vi "Arms Command.vi"(11 "Numeric":dbl) -> (1 "RightArmMotorCmd":dbl(graph), 2 "Right Arm Min Limit":bool, 3 "Right Arm Max Limit":bool, 4 "LeftArmMotorCmd":dbl(graph), 5 "Left Arm Max Limit":bool, 6 "Left Arm Min Limit":bool)   [LabVIEW 2017]
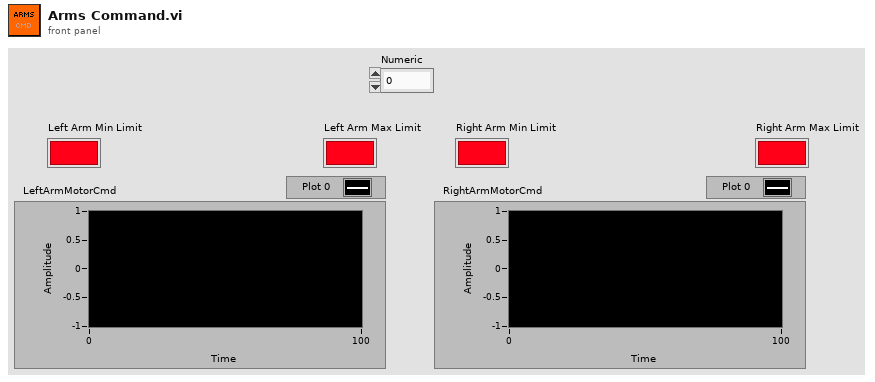
[diagram p1: front panel]
types:
  T1 = enum16{"initialize", "read", "write", "write all"}
  T2 = typedef "DioDisplayALB.ctl" = cluster{"DIO 0-LiftMinLimitSwitch":bool, "DIO 1-LiftMaxLimitSwitch":bool, "DIO 2-LiftArmMinLimitSwitch":bool, "DIO 3-LiftArmMaxLimitSwitch":bool, "DIO 4-RightArmMaxLimitSwitch":bool, "DIO 5-RightArmMinLimitSwitch":bool, "DIO 6-LeftArmMaxLimitSwitch":bool, "DIO 7-LeftArmMinLimitSwitch":bool, "DIO 8":bool, "DIO 9":bool}
  T3 = typedef "WPI_MotorControlDeviceRef.ctl" = cluster{"DeviceStatus":errorcluster, "Type":T4, "PWM":cluster{"PWM Channel":T5, "DeadBand":T6}, "CAN":cluster{"Device Number":u8, "SetOutput VI Ref":variant, "GetOutput VI Ref":variant, "Enable VI Ref":variant, "Disable VI Ref":variant, "Data":variant}, "Invert":bool, "DIO PWM":cluster{"PWM \"Enable\" Channel":T5, "DIOChannel":T7, "PWM Rate":dbl}}
  T4 = typedef "WPI_MotorControlType.ctl" = enum16{"PWM", "CAN", "DIO PWM"}
  T5 = typedef "FPGA_DIOPWMChannel.ctl" = enum8{"PWM 0", "PWM 1", "PWM 2", "PWM 3", "PWM 4", "PWM 5", "PWM 6", "PWM 7", "PWM 8", "PWM 9", "PWM MXP 0", "PWM MXP 1", "PWM MXP 2", "PWM MXP 3", "PWM MXP 4", "PWM MXP 5", "PWM MXP 6", "PWM MXP 7", "PWM MXP 8", "PWM MXP 9", "Invalid"}
  T6 = typedef "WPI_PWMDeadband.ctl" = cluster{"Name":string, "maxPositivePwm":i32, "minPositivePwm":i32, "centerPwm":i32, "maxNegativePwm":i32, "minNegativePwm":i32, "angularRange":u16}
  T7 = typedef "FPGA_DIOChannel.ctl" = enum8{"DIO 0", "DIO 1", "DIO 2", "DIO 3", "DIO 4", "DIO 5", "DIO 6", "DIO 7", "DIO 8", "DIO 9", "DIO MXP 0", "DIO MXP 1", "DIO MXP 2", "DIO MXP 3", "DIO MXP 4", "DIO MXP 5", "DIO MXP 6", "DIO MXP 7", "DIO MXP 8", "DIO MXP 9", "DIO MXP 10", "DIO MXP 11", "DIO MXP 12", "DIO MXP 13", "DIO MXP 14", "DIO MXP 15", "SPI Port CS1", "SPI Port CS2", "SPI Port CS3", "SPI Port MISO", "SPI Port MOSI", "Invalid"}
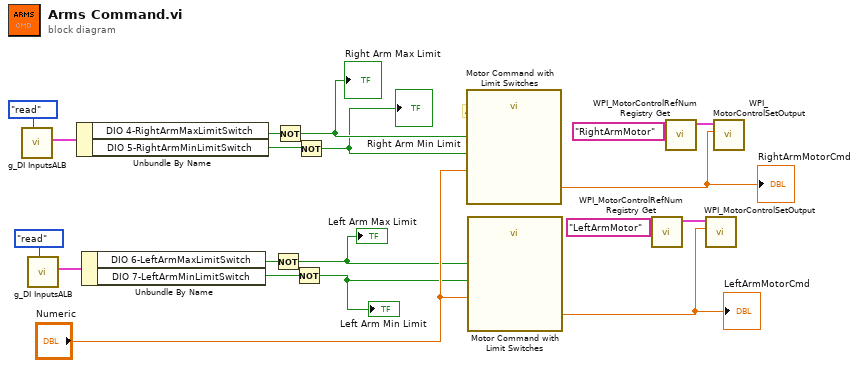
[diagram p0: block diagram]
diagram:
  # "Arms"
  n1 = call "g_DI InputsALB.vi"("Action"=T1."read") -> ("DI out"=w17:T2)  [unwired: 10 in]
  n2 = call "g_DI InputsALB.vi"("Action"=T1."read") -> ("DI out"=w18:T2)  [unwired: 10 in]
  n3 = Unbundle By Name(w17) -> ("DIO 4-RightArmMaxLimitSwitch"=w8:bool, "DIO 5-RightArmMinLimitSwitch"=w7:bool)
  n4 = Unbundle By Name(w18) -> ("DIO 6-LeftArmMaxLimitSwitch"=w6:bool, "DIO 7-LeftArmMinLimitSwitch"=w5:bool)
  n5 = Not(x=w6) -> (.not. x?=w14:bool)
  "Left Arm Max Limit" <- w14
  n6 = Not(x=w8) -> (.not. x?=w12:bool)
  "Right Arm Max Limit" <- w12
  n7 = Not(x=w5) -> (.not. x?=w13:bool)
  "Left Arm Min Limit" <- w13
  n8 = Not(x=w7) -> (.not. x?=w11:bool)
  "Right Arm Min Limit" <- w11
  n9 = call "Motor Command with Limit Switches.vi"("LowLimitSwitch"=w11, "MotorCommandIn"="Numeric", "HighLimitSwitch"=w12) -> (0:w9:dbl)
  "RightArmMotorCmd" <- w9
  n10 = call "Motor Command with Limit Switches.vi"("LowLimitSwitch"=w13, "MotorCommandIn"="Numeric", "HighLimitSwitch"=w14) -> (0:w10:dbl)
  "LeftArmMotorCmd" <- w10
  n11 = call <vilib>:"WPI_MotorControlRefNum Registry Get.vi"("refnum name"="LeftArmMotor") -> ("MotorControlDevRef"=w2:T3)  [unwired: 9 in, 1 out]
  n12 = call <vilib>:"WPI_MotorControlRefNum Registry Get.vi"("refnum name"="RightArmMotor") -> ("MotorControlDevRef"=w1:T3)  [unwired: 9 in, 1 out]
  n13 = call <vilib>:"WPI_MotorControlSetOutput.vi"("Output"=w10, "MotorControlDevRef"=w2) -> ()  [unwired: 7 in, 3 out]
  n14 = call <vilib>:"WPI_MotorControlSetOutput.vi"("Output"=w9, "MotorControlDevRef"=w1) -> ()  [unwired: 7 in, 3 out]
